vi "practica velocidad1.vi"() -> ()   [LabVIEW 2016]
panel:
  in  "aceleracion":dbl
  in  "velocidad":dbl
  out "distancia":dbl
  out "tiempo":i32
  in  "Boolean":bool
  in  "stop":bool
  out "Waveform Chart":cluster{"y":dbl, "y1":dbl}(graph)
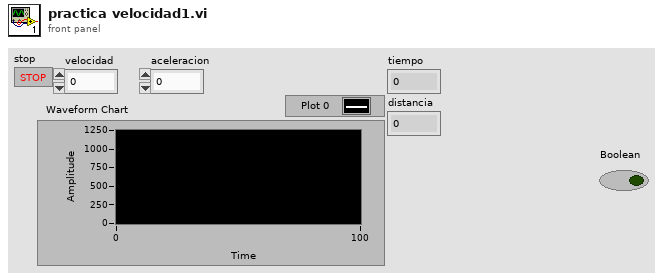
[diagram p1: front panel]
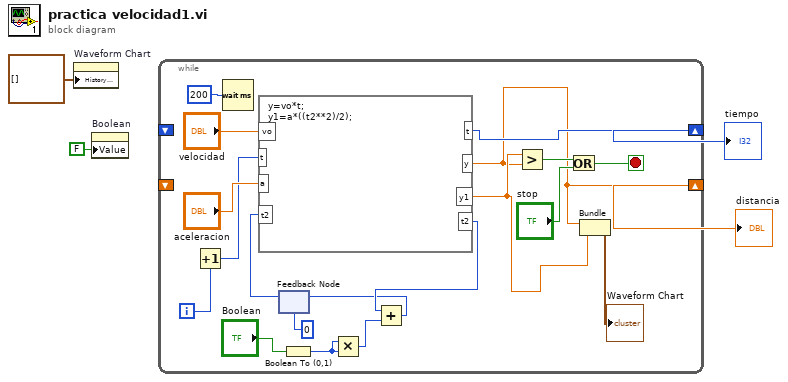
[diagram p0: block diagram]
diagram:
  n1 = property on="Waveform Chart" class="WFChart (strict)"("History Data"=cluster{"y":dbl, "y1":dbl}[] []) -> ()  [unwired: 2 in, 2 out]
  n2 = property on="Boolean" class="Bool (strict)"("Value"=FALSE ("Boolean")) -> ()  [unwired: 2 in, 2 out]
  n3 = while {
    shift-right: [w13] -> w4
    shift-left: _ -> [_]
    shift-right: [w9] -> w3
    shift-left: _ -> [_]
    i -> [w7]
    stop <- w19 stop-if-true
    n4 = Increment(x=w7) -> (x+1=w6:i32)
    n5 = Wait (ms)(milliseconds to wait=u32 200) -> ()  [unwired: 1 out]
    n6 = feedback #1(i16 0) -> (w14:i16)
    n7 = formula code="y=vo*t;\ny1=a*((t2**2)/2);"("t"=w6, "vo"="velocidad", "a"="aceleracion", "t2"=w14) -> ("y"=w9:dbl, "y1"=w10:dbl, "t2"=w17:i16, "t"=w13:i32)
    n8 = Boolean To (0,1)(Boolean="Boolean") -> (0, 1=w16:i16)
    n9 = Multiply(x=w16, y=w16) -> (x*y=w18:i16)
    n10 = Add(x=w17, y=w18) -> (x+y=w15:i16)
    n11 = feedback-in #1(w15) -> ()
    n12 = Greater?(x=w10, y=w9) -> (0:w21:bool)
    n13 = Or(x=w21, y="stop") -> (x .or. y?=w19:bool)
    n14 = Bundle("y"=w9, "y1"=w10) -> (→"Waveform Chart":cluster{"y":dbl, "y1":dbl})  [unwired: 1 in]
  }
  "tiempo" <- w4
  "distancia" <- w3
